vi "FieldBroadcaster.vi"   [LabVIEW 2025]
uses:
  ServerGlobalVariables.vi
types:
  T1 = cluster{"Troops":u32, "Owner":i32, "Mountain":bool, "City":bool, "General":bool, "Fog":bool}[][]
  T2 = cluster{"Troops":u32, "Owner":i32, "Mountain":bool, "City":bool, "General":bool, "Fog":bool}
  T3 = cluster{"Troops":u32, "Owner":i32, "Mountain":bool, "City":bool, "General":bool}[][]
  T4 = cluster{"Troops":u32, "Owner":i32, "Mountain":bool, "City":bool, "General":bool}
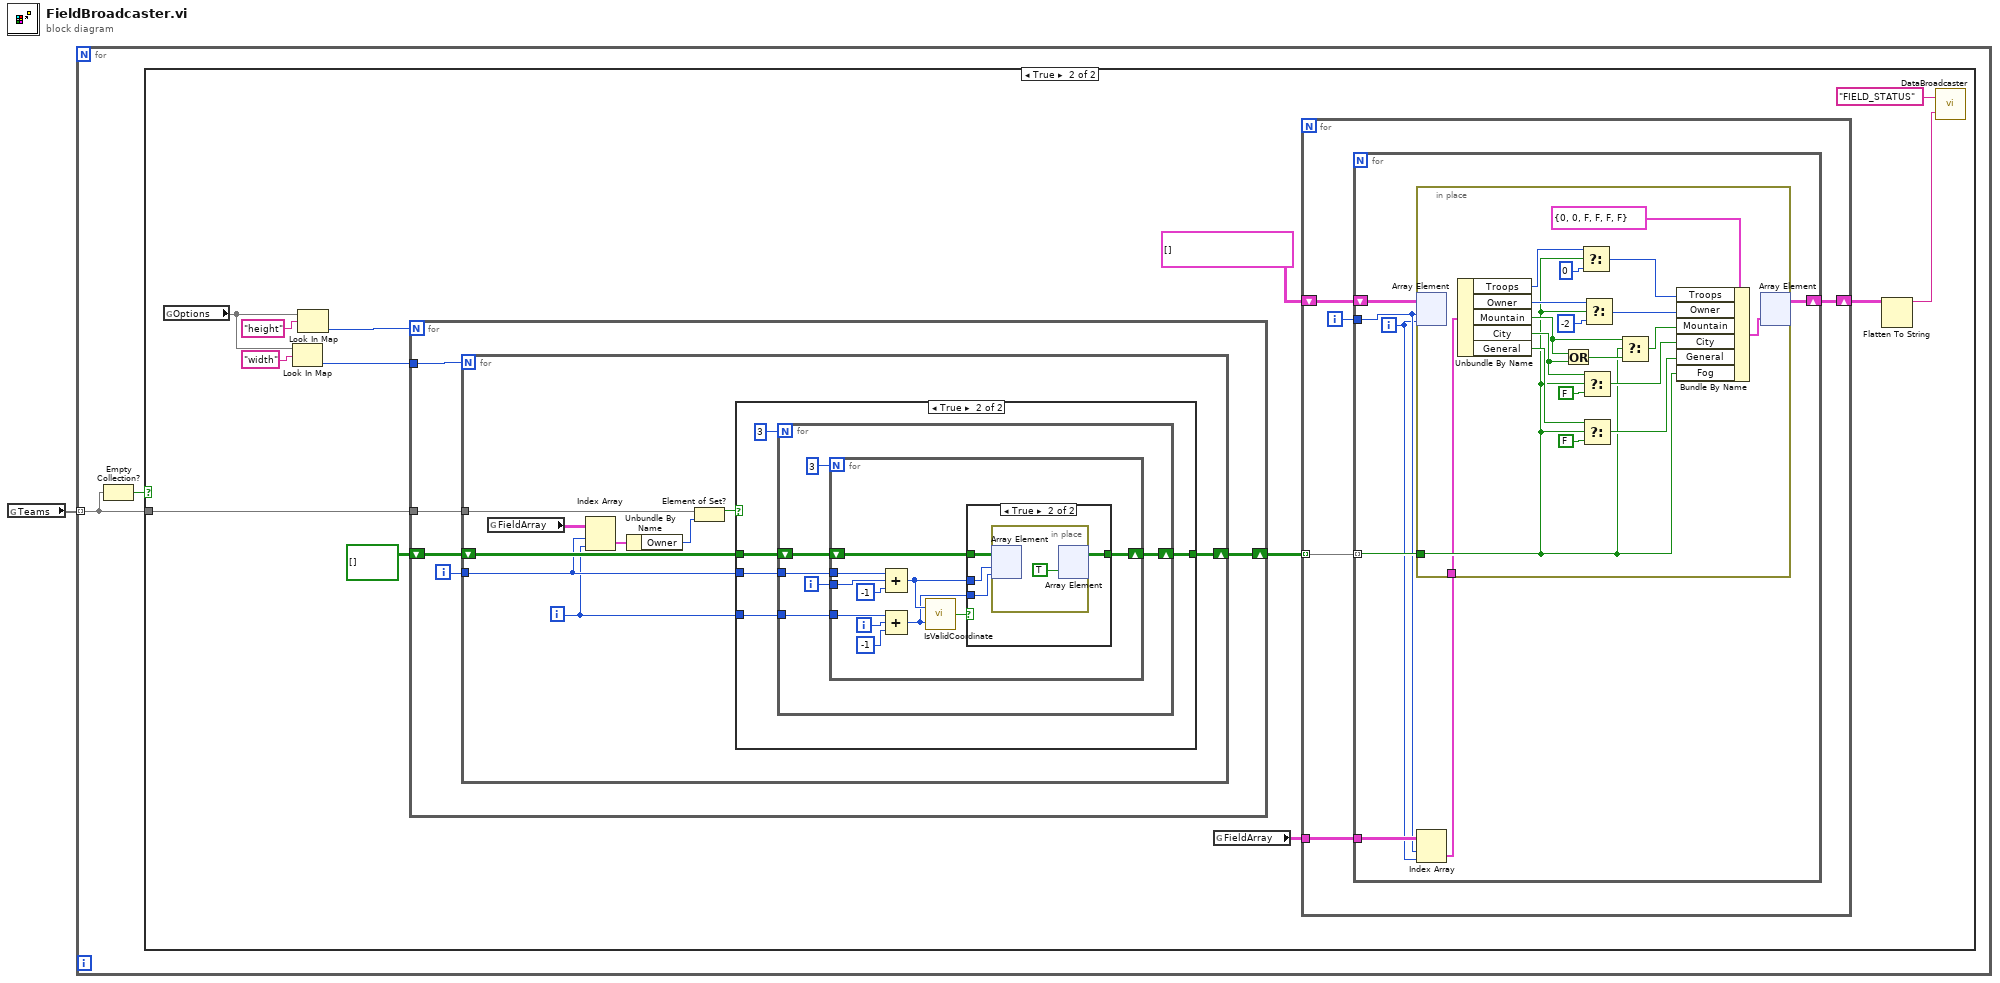
[diagram p0: block diagram]
diagram:
  n1 = global read "ServerGlobalVariables.vi" "Teams"() -> (w1:set{u32}[])
  n2 = for {
    tunnel: w1 -> [w2] mode=indexing
    n3 = Empty Collection?(1:w2) -> (0:w3:bool)
    n4 = case shown="True" w3 {
      tunnel: w2 -> [_ w11]
      frame False {
      }
      frame True {
        n5 = global read "ServerGlobalVariables.vi" "Options"() -> (w13:map{string, u32})
        n6 = Look In Map(map=w13, key="width") -> (value=w12:u32)  [unwired: 1 in, 1 out]
        n7 = Look In Map(map=w13, key="height") -> (value=w15:u32)  [unwired: 1 in, 1 out]
        n8 = for {
          N: w15 -> [_]
          tunnel: w12 -> [w52]
          shift-right: [w48] -> w9
          shift-left: bool[][] [] -> [w51]
          tunnel: w11 -> [w50]
          i -> [w49]
          n9 = for {
            N: w52 -> [_]
            shift-right: [w53] -> w48
            shift-left: w51 -> [w56]
            tunnel: w50 -> [w60]
            tunnel: w49 -> [w55]
            i -> [w54]
            n10 = global read "ServerGlobalVariables.vi" "FieldArray"() -> (w61:T3)
            n11 = Index Array(array=w61, index (row)=w55, index (col)=w54) -> (element=w59:T4)
            n12 = Unbundle By Name(w59) -> ("Owner"=w58:i32)
            n13 = Element of Set?(10:w58, 11:w60) -> (3:w57:bool)
            n14 = case shown="True" w57 {
              tunnel: w56 -> [w62 w66]
              tunnel: w55 -> [_ w65]
              tunnel: w54 -> [_ w64]
              tunnel: [w62 w63] -> w53
              frame False {
              }
              frame True {
                n15 = for {
                  N: 3 -> [_]
                  tunnel: w65 -> [w71]
                  tunnel: w64 -> [w70]
                  shift-right: [w68] -> w63
                  shift-left: w66 -> [w72]
                  i -> [w69]
                  n16 = for {
                    N: 3 -> [_]
                    tunnel: w71 -> [w84]
                    tunnel: w70 -> [w80]
                    tunnel: w69 -> [w83]
                    shift-right: [w74] -> w68
                    shift-left: w72 -> [w77]
                    i -> [w81]
                    n17 = Compound Arithmetic op=unknown(w84, w83, -1 ("value")) -> (w76:i32)
                    n18 = Compound Arithmetic op=ADD(w80, w81, -1 ("value")) -> (w75:i32)
                    n19 = call "IsValidCoordinate.vi"("Column"=w75, "Row"=w76) -> ("Valid"=w78:bool)
                    n20 = case shown="True" w78 {
                      tunnel: w77 -> [w85 w89]
                      tunnel: w76 -> [_ w88]
                      tunnel: w75 -> [_ w87]
                      tunnel: [w85 w86] -> w74
                      frame False {
                      }
                      frame True {
                        n21 = in-place {
                          n22 = in-place-array #1(w89, w88, w87) -> ()  [unwired: 1 out]
                          n23 = in-place-array #1(TRUE ("element")) -> (w86:bool[][])  [unwired: 2 out]
                        }
                      }
                    }
                  }
                }
              }
            }
          }
        }
        n24 = global read "ServerGlobalVariables.vi" "FieldArray"() -> (w5:T3)
        n25 = for {
          tunnel: w9 -> [w20] mode=indexing
          shift-right: [w19] -> w6
          shift-left: T1 [] ("FieldArray") -> [w21]
          tunnel: w5 -> [w17]
          i -> [w18]
          n26 = for {
            tunnel: w20 -> [w27] mode=indexing
            shift-right: [w26] -> w19
            shift-left: w21 -> [w28]
            tunnel: w18 -> [w24]
            tunnel: w17 -> [w25]
            i -> [w23]
            n27 = Index Array(array=w25, index (row)=w24, index (col)=w23) -> (element=w22:T4)
            n28 = in-place {
              in-place-border: w27 -> [w31]
              in-place-border: w22 -> [w30]
              n29 = in-place-array #2(w28, w24, w23) -> ()  [unwired: 1 out]
              n30 = Unbundle By Name(w30) -> ("Troops"=w42:u32, "Owner"=w41:i32, "Mountain"=w38:bool, "City"=w36:bool, "General"=w34:bool)
              n31 = Or(x=w38, y=w36) -> (x .or. y?=w37:bool)
              n32 = Select(t=w42, s=w31, f=u32 0) -> (s? t:f=w47:u32)
              n33 = Select(t=w36, s=w31, f=FALSE) -> (s? t:f=w44:bool)
              n34 = Select(t=w34, s=w31, f=FALSE) -> (s? t:f=w43:bool)
              n35 = Select(t=w41, s=w31, f=-2) -> (s? t:f=w46:i32)
              n36 = Select(t=w38, s=w31, f=w37) -> (s? t:f=w45:bool)
              n37 = Bundle By Name(cluster=T2 {"Troops"=0, "Owner"=0, "Mountain"=FALSE, "City"=FALSE, "General"=FALSE, "Fog"=FALSE} ("CellInfo"), "Troops"=w47, "Owner"=w46, "Mountain"=w45, "City"=w44, "General"=w43, "Fog"=w31) -> (w29:T2)
              n38 = in-place-array #2(w29) -> (w26:T1)  [unwired: 2 out]
            }
          }
        }
        n39 = Flatten To String(anything=w6) -> (data string=w7:string)  [unwired: 3 in, 2 out]
        n40 = call "DataBroadcaster.vi"("Data"=w7, "Action"="FIELD_STATUS") -> ()
      }
    }
  }
